vi "IECMemory.LoadDataMM6.vi"(0 "i ref in":refnum<vi>, 2 "MemDevInfo":T1, 3 "ms timeout (100)":i32=100, 5 "error in (no error)":errorcluster) -> (14 "i ref out":refnum<vi>, 17 "timed out":bool, 19 "error out":errorcluster)   [LabVIEW 2014, in "IECMemory.lvlib"]
uses:
  IECMemory.lvlib
  CS_Core/CSSystem/CoreDefs/CoreDefs.error_type.ctl
  CS_Core/CSSystem/CoreLib/CoreLib.lvlib
  CS_Lebit/LEBITDefs/LEBITDefs.MemDevInfo.ctl
  CS_Lebit/LEBITDefs/LEBITDefs.lvlib
  CS_Lebit/LEBITDefs/LEBITDefs.Memory.ctl
  CS_Lebit/LEBITDefs/LEBITDefs.Timetable.ctl
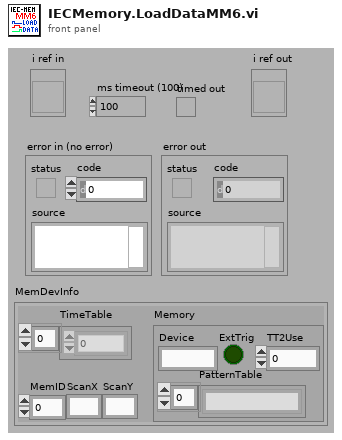
[diagram p1: front panel]
types:
  T1 = typedef "LEBITDefs.lvlib/LEBITDefs.MemDevInfo.ctl" = cluster{"TimeTable":T2, "Memory":T3, "MemID":i32, "ScanX":string, "ScanY":string}
  T2 = typedef "LEBITDefs.lvlib/LEBITDefs.Timetable.ctl" = dbl[]
  T3 = typedef "LEBITDefs.lvlib/LEBITDefs.Memory.ctl" = cluster{"Device":string, "ExtTrig":bool, "TT2Use":i32, "PatternTable":string[]}
  T4 = typedef "CoreDefs.error_type.ctl" = enum16{"no error", "can't load process", "can't unload process", "process does not exist", "can't install process", "can't remove process", "unknown function", "time out", "can't execute function", "duplicate queue name", "super not found", "caller queue invalid", "can't ping process", "unknown error", "VISA Error", "VISA timeout", "GPIB timeout", "GPIB error", "communication error", "data type mismatch", "can't read data from OPC server", "can't write data to OPC server", "OET error", "function not implemented", "process already exists", "invalid Shared Variable name", "error writing Shared Variable", "error reading Shared Variable", "invalid client name", "corrupt database", "unknown class", "call not authorized", "parameter out of range", "OET timeout: can't get data to modify", "invalid queue name", "requested operation incompatible with current state", "event undefined", "event disabled", "state undefined", "caller is not a friend", "EventBuilder: bad eventID", "EventBuilder: no DAQ devices", "a thread must not stop itself", "UNUSED ELEMENT4", "DiscArchiver: eventData incomplete", "DiscArchiver: eventData does not belong to run", "DiscArchiver: can't open file", "DiscArchiver: can't write to file", "DiscArchiver: available disc space low", "can't acquire semaphore", "error reading data from database", "notifier object is not existing", "can't register process", "can't unregister process", "illegal event type", "object disabled", "object already exists", "can't change state", "Instrument not found", "no connection to remote node", "invalid reference", "N/A", "UNUSED ELEMENT 1", "element not found", "illegal TCP/IP connection detected", "object does not exist", "invalid access ID", "unknown CS system", "invalid privilige", "unsupported data type", "unsupported server type", "IO server already exists", "Shared Variable already exists"}
  T5 = typedef "IECMemory.lvlib/IECMemory.i attribute.ctl" = cluster{"EndAddress":u32, "MemoryStatusBits":T6, "IEC Finished":bool, "Call Process":string, "Call Event":string}
  T6 = typedef "IECMemoryDriver.lvlib/Memory_Status.ctl" = bool[]
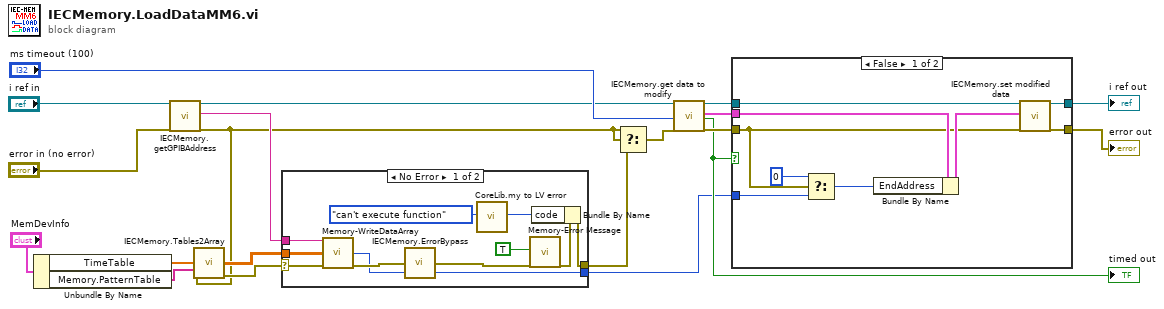
[diagram p0: block diagram]
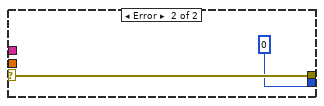
[diagram p2: hidden frame]
diagram:
  n1 = Unbundle By Name("MemDevInfo") -> ("TimeTable"=w5:T2, "Memory.PatternTable"=w4:string[])
  n2 = call "IECMemory.getGPIBAddress.vi"("i ref in"="i ref in", "error in (no error)"="error in (no error)") -> ("i ref out"=w14:refnum<vi>, "GPIBAddress"=w10:string, "error out"=w1:errorcluster)  [unwired: 14 in, 1 out]
  n3 = call "IECMemory.Tables2Array.vi"("Timing Num"=w5, "Logic"=w4, "error in (no error)"=w1) -> ("MemData"=w2:dbl[][], "error out"=w3:errorcluster)  [unwired: 11 in]
  n4 = case shown="No Error" w3 {
    selector: w3 -> [w26 w33]
    tunnel: [w28 w33] -> w7
    tunnel: [w22 u32 0] -> w9
    tunnel: w10 -> [w24 _]
    tunnel: w2 -> [w23 _]
    frame No Error {
      n5 = call "Memory-WriteDataArray.vi"("AddressStringIN"=w24, "MemoryTimingArray"=w23, "error in (no error)"=w26) -> ("EndAddress"=w22:i16, "error out"=w25:errorcluster)  [unwired: 11 in]
      n6 = call "IECMemory.ErrorBypass.vi"("error in (no error)"=w25) -> ("error out"=w21:errorcluster)  [unwired: 14 in]
      n7 = call "CoreLib.my to LV error.vi"("ErrorTypes"=CoreDefs.error_type."can't execute function") -> ("LV error code"=w27:i32)  [unwired: 17 in, 1 out]
      n8 = call "Memory-Error Message.vi"("add message to source"=TRUE, "error in (no error)"=w21) -> ("error out"=w29:errorcluster)  [unwired: 14 in, 3 out]
      n9 = Bundle By Name(cluster=w29, "code"=w27) -> (w28:errorcluster)
    }
    frame Error {
    }
  }
  n10 = Select(t=w1, s=w1, f=w7) -> (s? t:f=w8:errorcluster)
  n11 = call "IECMemory.get data to modify.vi"("i ref in"=w14, "ms timeout (10000)"="ms timeout (100)", "error in (no error)"=w8) -> ("i ref out"=w18:refnum<vi>, "i attribute"=w16:T5, "timed out"=w13:bool, "error out"=w17:errorcluster)  [unwired: 13 in]
  "timed out" <- w13
  n12 = case shown="False" w13 {
    tunnel: w18 -> [w38 w44]
    tunnel: [w40 w44] -> w12
    tunnel: [w39 w43] -> w11
    tunnel: w17 -> [w36 w43]
    tunnel: w16 -> [w42 _]
    tunnel: w9 -> [w34 _]
    frame False {
      n13 = Select(t=u32 0, s=w36, f=w34) -> (s? t:f=w41:u32)
      n14 = Bundle By Name(cluster=w42, "EndAddress"=w41) -> (w37:T5)
      n15 = call "IECMemory.set modified data.vi"("i ref in"=w38, "i attribute"=w37, "error in (no error)"=w36) -> ("i ref out"=w40:refnum<vi>, "error out"=w39:errorcluster)  [unwired: 15 in]
    }
    frame True {
    }
  }
  "error out" <- w11
  "i ref out" <- w12
